vi "Set inverted lines.vi"(8 "error in (no error)":errorcluster, 10 "Lines to invert":u8[](array[numeric]), 11 "TTL in":refnum<class "TTL.lvclass">) -> (0 "error out":errorcluster, 3 "TTL out":refnum<class "TTL.lvclass">)   [LabVIEW 2011, in "TTL.lvclass"]
uses:
  TTL.lvclass
  TTL.lvclass/TTL.ctl
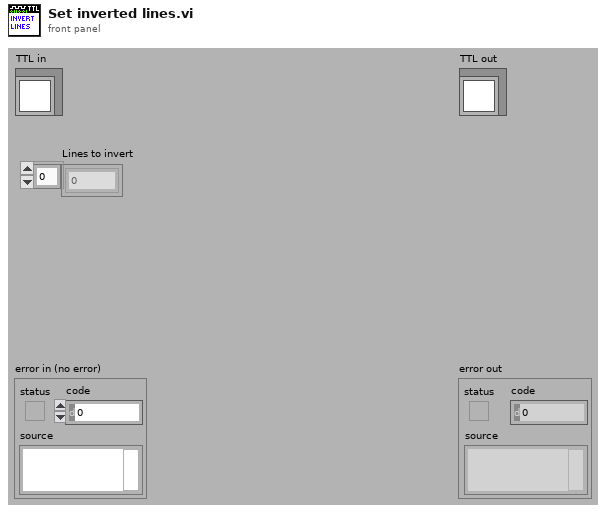
[diagram p1: front panel]
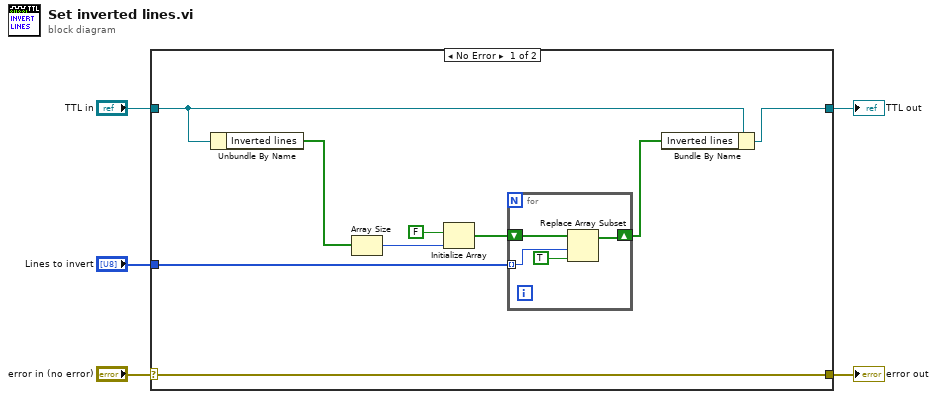
[diagram p0: block diagram]
diagram:
  n1 = case shown="No Error" "error in (no error)" {
    selector: "error in (no error)" -> [w14 w20]
    tunnel: [w14 w20] -> w4
    tunnel: [w11 w19] -> w2
    tunnel: "TTL in" -> [w10 w19]
    tunnel: "Lines to invert" -> [w9 _]
    frame No Error {
      n2 = Unbundle By Name(w10) -> ("Inverted lines"=w8:bool[])
      n3 = Array Size(array=w8) -> (size(s)=w7:i32)
      n4 = Initialize Array(FALSE, w7) -> (w12:bool[])
      n5 = for {
        shift-right: [w17] -> w6
        shift-left: w12 -> [w18]
        tunnel: w9 -> [w16] mode=indexing
        n6 = Replace Array Subset(array=w18, new element=TRUE ("new element/subarray"), index=w16) -> (w17:bool[])
      }
      n7 = Bundle By Name(cluster=w10, "Inverted lines"=w6) -> (w11:refnum<class "TTL.lvclass">)
    }
    frame Error {
    }
  }
  "error out" <- w4
  "TTL out" <- w2
